vi "log analysis_gps.vi"() -> ()   [LabVIEW 2018] (continued)
02008000,d426,15824;INSUFFICIENT_OBS,NONE,0.000000000,0.000000000,0.000000000,0.0,0.000000000,0.000000000,\"\",0,0,0,0,00,00,00,00*bcb2c0dd\n\tsystem status\tnormal 2 28.100000 0 0\trobot status\t274.912306\t76.948987\t9.582700\t-0.292788\t1.088000\t-30.605308\t0.352000\t0.058000\n\t\n15:22:58.5\tlog_raw\tgps_raw\t#DUALANTENNAHEADINGA,USB3,0,49.0,FINESTEERING,2107,282196.500,02008000,d426,15824;SOL_COMPUTED,NARROW_FLOAT,-1.000000000,119.397575378,5.704736233,0.0,360.000000000,180.000000000,\"631T\",17,6,6,5,04,00,20,03*618b4b70\n\tsystem status\tnormal 2 28.000000 0 0\trobot status\t275.029815\t76.849491\t9.589700\t-0.210069\t0.973059\t-30.986366\t0.294000\t-0.025000\n\t\n15:22:59.0\tlog_raw\tgps_raw\t\tsystem status\tnormal 2 28.000000 0 0\trobot status\t275.145656\t76.747954\t9.596500\t-0.145332\t0.980754\t-31.500751\t0.356000\t0.072000\n\t\n15:22:59.5\tlog_raw\tgps_raw\t#DUALANTENNAHEADINGA,USB3,0,52.0,FINESTEERING,2107,282197.500,02008000,d426,15824;SOL_COMPUTED,NARROW_FLOAT,-1.000000000,59.046657562,-17.785888672,0.0,166.409759521,180.000000000,\"631T\",16,7,7,5,04,00,20,03*00118b7f\n\tsystem status\tnormal 2 28.000000 0 0\trobot status\t275.261842\t76.668742\t9.599000\t-0.003183\t0.966963\t-31.967987\t0.353000\t0.059000\n\t\n15:23:00.0\tlog_raw\tgps_raw\t#DUALANTENNAHEADINGA,USB3,0,52.0,FINESTEERING,2107,282198.000,02008000,d426,15824;SOL_COMPUTED,NARROW_FLOAT,-1.000000000,59.079334259,-18.122131348,0.0,167.196258545,180.000000000,\"631T\",16,7,7,5,04,00,20,03*485efbcb\n\tsystem status\tnormal 2 28.000000 0 0\trobot status\t275.377702\t76.588966\t9.600500\t-0.044192\t1.138417\t-32.357221\t0.252000\t-0.086000\n\t\n15:23:00.5\tlog_raw\tgps_raw\t#DUALANTENNAHEADINGA,USB3,0,50.0,FINESTEERING,2107,282198.500,02000000,d426,15824;SOL_COMPUTED,NARROW_FLOAT,-1.000000000,72.630279541,-6.125091553,0.0,217.219696045,180.000000000,\"631T\",16,8,8,5,04,00,20,03*03cea49d\n\tsystem status\tnormal 2 28.000000 0 0\trobot status\t275.489352\t76.505166\t9.604900\t-0.094622\t1.328061\t-32.726048\t0.293000\t-0.019000\n\t\n15:23:01.0\tlog_raw\tgps_raw\t#DUALANTENNAHEADINGA,USB3,0,50.0,FINESTEERING,2107,282199.000,02000000,d426,15824;SOL_COMPUTED,NARROW_FLOAT,-1.000000000,72.616973877,-5.097595215,0.0,218.517272949,180.000000000,\"631T\",18,8,8,5,04,00,20,03*278af582\n\tsystem status\tnormal 2 28.100000 0 0\trobot status\t275.601783\t76.419379\t9.608400\t-0.185416\t1.532796\t-32.964629\t0.298000\t-0.002000\n\t\n15:23:01.5\tlog_raw\tgps_raw\t#DUALANTENNAHEADINGA,USB3,0,51.0,FINESTEERING,2107,282199.500,02000000,d426,15824;INSUFFICIENT_OBS,NONE,0.000000000,0.000000000,0.000000000,0.0,0.000000000,0.000000000,\"\",0,0,0,0,00,00,00,00*6fb354b0\n\tsystem status\tnormal 2 28.000000 0 0\trobot status\t275.709417\t76.334818\t9.610400\t-0.145091\t1.698029\t-33.199566\t0.306000\t0.004000\n\t\n15:23:02.0\tlog_raw\tgps_raw\t\tsystem status\tnormal 2 28.100000 0 0\trobot status\t275.819505\t76.245723\t9.612400\t-0.060143\t1.689752\t-33.413572\t0.300000\t0.007000\n\t\n15:23:02.5\tlog_raw\tgps_raw\t#DUALANTENNAHEADINGA,USB3,0,51.5,FINESTEERING,2107,282200.500,02000000,d426,15824;INSUFFICIENT_OBS,NONE,0.000000000,0.000000000,0.000000000,0.0,0.000000000,0.000000000,\"\",0,0,0,0,00,00,00,00*ba5dc1a6\n\tsystem status\tnormal 2 28.100000 0 0\trobot status\t275.926001\t76.142312\t9.618400\t0.095795\t1.531020\t-33.633287\t0.295000\t0.013000\n\t\n15:23:03.0\tlog_raw\tgps_raw\t#DUALANTENNAHEADINGA,USB3,0,51.5,FINESTEERING,2107,282201.000,02000000,d426,15824;INSUFFICIENT_OBS,NONE,0.000000000,0.000000000,0.000000000,0.0,0.000000000,0.000000000,\"\",0,0,0,0,00,00,00,00*13cea2a1\n\tsystem status\tnormal 2 28.100000 0 0\trobot status\t276.031687\t76.036831\t9.624600\t0.090096\t1.284244\t-33.885924\t0.303000\t0.003000\n\t\n15:23:03.5\tlog_raw\tgps_raw\t#DUALANTENNAHEADINGA,USB3,0,53.0,FINESTEERING,2107,282201.500,02000000,d426,15824;INSUFFICIENT_OBS,NONE,0.000000000,0.000000000,0.000000000,0.0,0.000000000,0.000000000,\"\",0,0,0,0,00,00,00,00*311e64df\n\tsystem status\tnormal 2 28.100000 0 0\trobot status\t276.138696\t75.928855\t9.630700\t-0.035823\t1.113523\t-34.018971\t0.301000\t0.004000\n\t\n15:23:04.0\tlog_raw\tgps_raw\t#INSPVAXA,USB3,0,53.0,FINESTEERING,2107,282202.050,02000000,471d,15824;INS_ALIGNMENT_COMPLETE,INS_RTKFIXED,37.37081327952,126.72395394538,9.6368,22.3000,-0.2188,0.2169,0.0119,-0.186356861,0.873042918,124.050200417,0.5705,0.3686,0.6665,0.1331,0.1050,0.0820,0.1461,0.1508,4.9895,0f000001,0*b1c71fb3\n\tsystem status\tnormal 2 28.100000 0 0\trobot status\t276.261764\t75.807130\t9.636800\t-0.186357\t0.873043\t-34.050200\t0.298000\t0.025000\n\t\n15:23:04.5\tlog_raw\tgps_raw\t#DUALANTENNAHEADINGA,USB3,0,53.0,FINESTEERING,2107,282202.500,02000000,d426,15824;INSUFFICIENT_OBS,NONE,0.000000000,0.000000000,0.000000000,0.0,0.000000000,0.000000000,\"\",0,0,0,0,00,00,00,00*e4587ba4\n\tsystem status\tnormal 2 28.100000 0 0\trobot status\t276.364792\t75.742837\t9.636100\t-0.196635\t0.813843\t-34.065150\t0.302000\t0.016000\n\t\n15:23:05.0\tlog_raw\tgps_raw\t\tsystem status\tnormal 2 28.100000 0 0\trobot status\t276.481226\t75.668811\t9.635600\t-0.212412\t0.914728\t-33.926312\t0.295000\t0.037000\n\t\n15:23:05.5\tlog_raw\tgps_raw\t#DUALANTENNAHEADINGA,USB3,0,52.5,FINESTEERING,2107,282203.500,02000000,d426,15824;INSUFFICIENT_OBS,NONE,0.000000000,0.000000000,0.000000000,0.0,0.000000000,0.000000000,\"\",0,0,0,0,00,00,00,00*55500259\n\tsystem status\tnormal 2 28.000000 0 0\trobot status\t276.590081\t75.590259\t9.636200\t-0.255814\t1.160317\t-33.428711\t0.308000\t0.019000\n\t\n15:23:06.0\tlog_raw\tgps_raw\t#DUALANTENNAHEADINGA,USB3,0,52.5,FINESTEERING,2107,282204.000,02000000,d426,15824;INSUFFICIENT_OBS,NONE,0.000000000,0.000000000,0.000000000,0.0,0.000000000,0.000000000,\"\",0,0,0,0,00,00,00,00*8d3e59e9\n\tsystem status\tnormal 2 27.900000 0 0\trobot status\t276.699631\t75.510509\t9.636500\t-0.377307\t1.263158\t-32.842107\t0.247000\t0.122000\n\t\n15:23:06.5\tlog_raw\tgps_raw\t#DUALANTENNAHEADINGA,USB3,0,51.0,FINESTEERING,2107,282204.500,02000000,d426,15824;INSUFFICIENT_OBS,NONE,0.000000000,0.000000000,0.000000000,0.0,0.000000000,0.000000000,\"\",0,0,0,0,00,00,00,00*0f0729d4\n\tsystem status\tnormal 2 27.800000 0 0\trobot status\t276.809810\t75.428563\t9.637300\t-0.231259\t1.268189\t-32.036520\t0.321000\t-0.003000\n\t\n15:23:07.0\tlog_raw\tgps_raw\t#DUALANTENNAHEADINGA,USB3,0,51.0,FINESTEERING,2107,282205.000,02000000,d426,15824;INSUFFICIENT_OBS,NONE,0.000000000,0.000000000,0.000000000,0.0,0.000000000,0.000000000,\"\",0,0,0,0,00,00,00,00*a6944ad3\n\tsystem status\tnormal 2 27.800000 0 0\trobot status\t276.920112\t75.348048\t9.638800\t-0.239719\t1.316167\t-31.223244\t0.236000\t0.118000\n\t\n15:23:07.5\tlog_raw\tgps_raw\t#INSPVAXA,USB3,0,53.0,FINESTEERING,2107,282205.550,02000000,471d,15824;INS_ALIGNMENT_COMPLETE,INS_RTKFIXED,37.37080836161,126.72396276793,9.6416,22.3000,-0.1860,0.2071,0.0131,-0.386237620,1.395044510,120.415786575,0.4755,0.3044,0.5933,0.1227,0.0990,0.0774,0.1450,0.1497,4.9912,0f000001,0*671127a5\n\tsystem status\tnormal 2 27.800000 0 0\trobot status\t277.043251\t75.261292\t9.641600\t-0.386238\t1.395045\t-30.415787\t0.255000\t0.098000\n\t\n15:23:08.0\tlog_raw\tgps_raw\t#DUALANTENNAHEADINGA,USB3,0,53.0,FINESTEERING,2107,282206.000,02000000,d426,15824;INSUFFICIENT_OBS,NONE,0.000000000,0.000000000,0.000000000,0.0,0.000000000,0.000000000,\"\",0,0,0,0,00,00,00,00*e9703f6f\n\tsystem status\tnormal 2 27.900000 0 0\trobot status\t277.146093\t75.189189\t9.643900\t-0.464725\t1.386082\t-29.903743\t0.334000\t-0.013000\n\t\n15:23:08.5\tlog_raw\tgps_raw\t\tsystem status\tnormal 2 27.900000 0 0\trobot status\t277.259307\t75.112413\t9.646000\t-0.468117\t1.652568\t-29.339662\t0.270000\t0.070000\n\t\n15:23:09.0\tlog_raw\tgps_raw\t#INSPVAXA,USB3,0,52.0,FINESTEERING,2107,282207.050,02000000,471d,15824;INS_ALIGNMENT_COMPLETE,INS_RTKFIXED,37.37080624605,126.72396663060,9.6483,22.3000,-0.1799,0.2155,-0.0033,-0.382267918,1.666666307,118.913486054,0.4622,0.2990,0.5698,0.1222,0.0981,0.0770,0.1443,0.1494,4.9912,0f000001,0*412cbbed\n\tsystem status\tnormal 2 27.900000 0 0\trobot status\t277.385400\t75.026486\t9.648300\t-0.382268\t1.666666\t-28.913486\t0.315000\t-0.016000\n\t\n15:23:09.5\tlog_raw\tgps_raw\t#INSPVAXA,USB3,0,52.5,FINESTEERING,2107,282207.550,02000000,471d,15824;INS_ALIGNMENT_COMPLETE,INS_RTKFIXED,37.37080553452,126.72396795365,9.6521,22.3000,-0.1872,0.2206,-0.0051,-0.332963269,1.523153610,118.680008658,0.4622,0.2990,0.5698,0.1222,0.0981,0.0770,0.1443,0.1494,4.9912,0f000001,0*ceea6f3f\n\tsystem status\tnormal 2 28.000000 0 0\trobot status\t277.502593\t74.947513\t9.652100\t-0.332963\t1.523154\t-28.680009\t0.216000\t0.117000\n\t\n15:23:10.0\tlog_raw\tgps_raw\t#DUALANTENNAHEADINGA,USB3,0,52.5,FINESTEERING,2107,282208.000,02000000,d426,15824;INSUFFICIENT_OBS,NONE,0.000000000,0.000000000,0.000000000,0.0,0.000000000,0.000000000,\"\",0,0,0,0,00,00,00,00*6ec42887\n\tsystem status\tnormal 2 28.000000 0 0\trobot status\t277.607938\t74.876095\t9.655100\t-0.292418\t1.472958\t-28.591290\t0.334000\t-0.074000\n\t\n15:23:10.5\tlog_raw\tgps_raw\t\tsystem status\tnormal 2 28.000000 0 0\trobot status\t277.716428\t74.786283\t9.660500\t-0.341323\t1.522114\t-28.516894\t0.278000\t0.020000\n\t\n15:23:11.0\tlog_raw\tgps_raw\t\tsystem status\tnormal 2 28.100000 0 0\trobot status\t277.824920\t74.695483\t9.666100\t-0.489851\t1.492802\t-28.563133\t0.288000\t0.002000\n\t\n15:23:11.5\tlog_raw\tgps_raw\t#DUALANTENNAHEADINGA,USB3,0,53.0,FINESTEERING,2107,282209.500,02000000,d426,15824;SOL_COMPUTED,L1_FLOAT,-1.000000000,126.771110535,-42.657562256,0.0,360.000000000,180.000000000,\"631T\",15,6,6,5,04,00,20,03*5e6f8f1e\n\tsystem status\tnormal 2 28.100000 0 0\trobot status\t277.950579\t74.626425\t9.668500\t-0.427356\t1.503272\t-28.579089\t0.296000\t-0.011000\n\t\n15:23:12.0\tlog_raw\tgps_raw\t\tsystem status\tnormal 2 28.100000 0 0\trobot status\t278.077777\t74.556796\t9.671200\t-0.353609\t1.534540\t-28.611370\t0.297000\t-0.008000\n\t\n15:23:12.5\tlog_raw\tgps_raw\t#INSPVAXA,USB3,0,46.5,FINESTEERING,2107,282210.550,02000000,471d,15824;INS_ALIGNMENT_COMPLETE,INS_RTKFIXED,37.37080130132,126.72397594412,9.6761,22.3000,-0.1788,0.2268,0.0030,-0.286685420,1.503985922,118.659616564,0.4924,0.3183,0.5916,0.1238,0.0973,0.0785,0.1441,0.1495,4.9922,0f000001,0*a986a7a1\n\tsystem status\tnormal 2 28.100000 0 0\trobot status\t278.210376\t74.477669\t9.676100\t-0.286685\t1.503986\t-28.659617\t0.298000\t-0.010000\n\t\n15:23:13.0\tlog_raw\tgps_raw\t#INSPVAXA,USB3,0,46.5,FINESTEERING,2107,282211.050,02000000,471d,15824;INS_ALIGNMENT_COMPLETE,INS_RTKFIXED,37.37080065460,126.72397731700,9.6819,22.3000,-0.1828,0.2291,0.0069,-0.471563317,1.301185162,118.765096011,0.4785,0.3076,0.5799,0.1215,0.0954,0.0779,0.1439,0.1491,4.9928,0f000001,0*2dcee279\n\tsystem status\tnormal 2 28.000000 0 0\trobot status\t278.331984\t74.405889\t9.681900\t-0.471563\t1.301185\t-28.765096\t0.298000\t-0.016000\n\t\n15:23:13.5\tlog_raw\tgps_raw\t#INSPVAXA,USB3,0,49.5,FINESTEERING,2107,282211.550,02000000,471d,15824;INS_ALIGNMENT_COMPLETE,INS_RTKFIXED,37.37079998486,126.72397867623,9.6862,22.3000,-0.1762,0.2152,0.0021,-0.525326899,1.337901633,118.895801631,0.4785,0.3076,0.5799,0.1215,0.0954,0.0779,0.1439,0.1491,4.9928,0f000001,0*f623f6b1\n\tsystem status\tnormal 2 28.100000 0 0\trobot status\t278.452382\t74.331555\t9.686200\t-0.525327\t1.337902\t-28.895802\t0.297000\t-0.027000\n\t\n15:23:14.0\tlog_raw\tgps_raw\t\tsystem status\tnormal 2 28.100000 0 0\trobot status\t278.560279\t74.263479\t9.689600\t-0.578283\t1.310440\t-29.026777\t0.307000\t-0.012000\n\t\n15:23:14.5\tlog_raw\tgps_raw\t#INSPVAXA,USB3,0,48.0,FINESTEERING,2107,282212.550,02000000,471d,15824;INS_ALIGNMENT_COMPLETE,INS_RTKFIXED,37.37079858565,126.72398137805,9.6949,22.3000,-0.1865,0.2376,0.0037,-0.452411122,1.244077399,119.281089900,0.4696,0.3015,0.5709,0.1202,0.0946,0.0776,0.1439,0.1489,4.9934,0f000001,0*f2809ec3\n\tsystem status\tnormal 2 28.100000 0 0\trobot status\t278.691705\t74.176256\t9.694900\t-0.452411\t1.244077\t-29.281090\t0.298000\t-0.029000\n\t\n15:23:15.0\tlog_raw\tgps_raw\t#INSPVAXA,USB3,0,48.0,FINESTEERING,2107,282213.050,02000000,471d,15824;INS_ALIGNMENT_COMPLETE,INS_RTKFIXED,37.37079782312,126.72398277607,9.6996,22.3000,-0.1874,0.2360,0.0136,-0.341636601,1.253165011,119.484687507,0.4696,0.3015,0.5709,0.1202,0.0946,0.0776,0.1439,0.1489,4.9934,0f000001,0*32ae8dd5\n\tsystem status\tnormal 2 28.000000 0 0\trobot status\t278.815539\t74.091623\t9.699600\t-0.341637\t1.253165\t-29.484688\t0.300000\t-0.023000\n\t\n15:23:15.5\tlog_raw\tgps_raw\t#INSPVAXA,USB3,0,52.0,FINESTEERING,2107,282213.550,02000000,471d,15824;INS_ALIGNMENT_COMPLETE,INS_RTKFIXED,37.37079696943,126.72398406821,9.7061,22.3000,-0.1973,0.2288,0.0187,-0.230921805,1.180153263,119.768927864,0.4696,0.3015,0.5709,0.1202,0.0946,0.0776,0.1439,0.1489,4.9934,0f000001,0*21be5dd7\n\tsystem status\tnormal 2 28.000000 0 0\trobot status\t278.929995\t73.996872\t9.706100\t-0.230922\t1.180153\t-29.768928\t0.303000\t-0.009000\n\t\n15:23:16.0\tlog_raw\tgps_raw\t#INSPVAXA,USB3,0,52.0,FINESTEERING,2107,282214.050,02000000,471d,15824;INS_ALIGNMENT_COMPLETE,INS_RTKFIXED,37.37079609402,126.72398538509,9.7128,22.3000,-0.1984,0.2265,0.0093,-0.318894921,1.159811562,120.132243890,0.4696,0.3015,0.5709,0.1202,0.0946,0.0776,0.1439,0.1489,4.9934,0f000001,0*fc389eb4\n\tsystem status\tnormal 2 28.100000 0 0\trobot status\t279.046642\t73.899711\t9.712800\t-0.318895\t1.159812\t-30.132244\t0.277000\t-0.051000\n\t\n15:23:16.5\tlog_raw\tgps_raw\t\tsystem status\tnormal 2 28.000000 0 0\trobot status\t279.147927\t73.812646\t9.718900\t-0.463860\t1.163408\t-30.444630\t0.301000\t-0.026000\n\t\n15:23:17.0\tlog_raw\tgps_raw\t#INSPVAXA,USB3,0,52.0,FINESTEERING,2107,282215.050,02000000,471d,15824;INS_ALIGNMENT_COMPLETE,INS_RTKFIXED,37.37079433087,126.72398790668,9.7264,22.3000,-0.2059,0.2196,0.0017,-0.257763882,1.185688863,120.911498528,0.5642,0.3665,0.6560,0.1320,0.1043,0.0817,0.1458,0.1507,4.9969,0f000001,0*cb6b0c5a\n\tsystem status\tnormal 2 28.000000 0 0\trobot status\t279.270000\t73.704021\t9.726400\t-0.257764\t1.185689\t-30.911499\t0.331000\t0.039000\n\t\n15:23:17.5\tlog_raw\tgps_raw\t#INSPVAXA,USB3,0,51.0,FINESTEERING,2107,282215.550,02000000,471d,15824;INS_ALIGNMENT_COMPLETE,INS_RTKFIXED,37.37079367366,126.72398934399,9.7308,22.3000,-0.1996,0.2242,0.0120,-0.145309566,1.145371194,121.351414848,0.5642,0.3665,0.6560,0.1320,0.1043,0.0817,0.1458,0.1507,4.9969,0f000001,0*eab453aa\n\tsystem status\tnormal 2 28.000000 0 0\trobot status\t279.397315\t73.631077\t9.730800\t-0.145310\t1.145371\t-31.351415\t0.343000\t0.047000\n\t\n15:23:18.0\tlog_raw\tgps_raw\t#INSPVAXA,USB3,0,50.0,FINESTEERING,2107,282216.050,02008000,471d,15824;INS_ALIGNMENT_COMPLETE,INS_RTKFIXED,37.37079301498,126.72399074721,9.7351,22.3000,-0.2016,0.2239,0.0141,-0.200785279,1.162503620,121.722794866,0.5181,0.3306,0.6284,0.1253,0.0993,0.0793,0.1452,0.1498,4.9985,0f000001,0*bb6b6e1a\n\tsystem status\tnormal 2 28.100000 0 0\trobot status\t279.521610\t73.557970\t9.735100\t-0.200785\t1.162504\t-31.722795\t0.350000\t0.062000\n\t\n15:23:18.5\tlog_raw\tgps_raw\t#INSPVAXA,USB3,0,50.0,FINESTEERING,2107,282216.550,02008000,471d,15824;INS_ALIGNMENT_COMPLETE,INS_RTKFIXED,37.37079227472,126.72399206413,9.7382,22.3000,-0.1946,0.2230,0.0198,-0.317684959,1.282586608,122.063744608,0.5181,0.3306,0.6284,0.1253,0.0993,0.0793,0.1452,0.1498,4.9985,0f000001,0*e6f737e3\n\tsystem status\tnormal 2 28.100000 0 0\trobot status\t279.638260\t73.475808\t9.738200\t-0.317685\t1.282587\t-32.063745\t0.299000\t-0.007000\n\t\n15:23:19.0\tlog_raw\tgps_raw\t#INSPVAXA,USB3,0,50.0,FINESTEERING,2107,282217.050,02008000,471d,15824;INS_ALIGNMENT_COMPLETE,INS_RTKFIXED,37.37079150006,126.72399338506,9.7418,22.3000,-0.1973,0.2143,0.0166,-0.258493900,1.347892765,122.299122592,0.4919,0.3126,0.6073,0.1228,0.0982,0.0779,0.1450,0.1495,4.9999,0f000001,0*de2ea87f\n\tsystem status\tnormal 2 28.100000 0 0\trobot status\t279.755266\t73.389829\t9.741800\t-0.258494\t1.347893\t-32.299123\t0.297000\t-0.005000\n\t\n15:23:19.5\tlog_raw\tgps_raw\t\tsystem status\tnormal 2 28.100000 0 0\trobot status\t279.855684\t73.313958\t9.747600\t-0.193916\t1.492610\t-32.596087\t0.298000\t-0.002000\n\t\n15:23:20.0\tlog_raw\tgps_raw\t\tsystem status\tnormal 2 28.000000 0 0\trobot status\t279.966679\t73.228541\t9.754600\t-0.196447\t1.616666\t-32.901459\t0.292000\t-0.010000\n\t\n15:23:20.5\tlog_raw\tgps_raw\t#INSPVAXA,USB3,0,51.5,FINESTEERING,2107,282218.550,02008000,471d,15824;INS_ALIGNMENT_COMPLETE,INS_RTKFIXED,37.37078915904,126.72399716309,9.7610,22.3000,-0.2130,0.2098,0.0170,-0.292581924,1.665037995,123.167578818,0.4769,0.3037,0.5912,0.1221,0.0981,0.0771,0.1448,0.1493,5.0010,0f000001,0*5a89842f\n\tsystem status\tnormal 2 28.100000 0 0\trobot status\t280.089918\t73.130001\t9.761000\t-0.292582\t1.665038\t-33.167579\t0.297000\t-0.001000\n\t\n15:23:21.0\tlog_raw\tgps_raw\t#INSPVAXA,USB3,0,51.5,FINESTEERING,2107,282219.050,02008000,471d,15824;INS_ALIGNMENT_COMPLETE,INS_RTKFIXED,37.37078832063,126.72399842807,9.7659,22.3000,-0.2077,0.2129,0.0166,-0.240249053,1.576876220,123.403306266,0.4687,0.2996,0.5787,0.1217,0.0981,0.0767,0.1445,0.1492,5.0017,0f000001,0*d445f717\n\tsystem status\tnormal 2 28.100000 0 0\trobot status\t280.201968\t73.036946\t9.765900\t-0.240249\t1.576876\t-33.403306\t0.300000\t0.000000\n\t\n15:23:21.5\tlog_raw\tgps_raw\t#INSPVAXA,USB3,0,52.5,FINESTEERING,2107,282219.550,02008000,471d,15824;INS_ALIGNMENT_COMPLETE,INS_RTKFIXED,37.37078751914,126.72399965144,9.7712,22.3000,-0.2065,0.2085,0.0140,-0.281116396,1.447393421,123.657865027,0.4687,0.2996,0.5787,0.1217,0.0981,0.0767,0.1445,0.1492,5.0017,0f000001,0*13bb7dd6\n\tsystem status\tnormal 2 28.000000 0 0\trobot status\t280.310332\t72.947989\t9.771200\t-0.281116\t1.447393\t-33.657865\t0.300000\t0.003000\n\t\n15:23:22.0\tlog_raw\tgps_raw\t#INSPVAXA,USB3,0,52.5,FINESTEERING,2107,282220.050,02008000,471d,15824;INS_ALIGNMENT_COMPLETE,INS_RTKFIXED,37.37078669426,126.72400086844,9.7773,22.3000,-0.1998,0.2016,0.0200,-0.389870934,1.544632790,123.892841428,0.4687,0.2996,0.5787,0.1217,0.0981,0.0767,0.1445,0.1492,5.0017,0f000001,0*0724934d\n\tsystem status\tnormal 2 28.100000 0 0\trobot status\t280.418132\t72.856437\t9.777300\t-0.389871\t1.544633\t-33.892841\t0.298000\t0.008000\n\t\n15:23:22.5\tlog_raw\tgps_raw\t#INSPVAXA,USB3,0,45.0,FINESTEERING,2107,282220.550,02000000,471d,15824;INS_ALIGNMENT_COMPLETE,INS_RTKFIXED,37.37078572061,126.72400205426,9.7874,22.3000,-0.2160,0.2146,0.0148,-0.304638903,1.496803288,124.054451305,0.4687,0.2996,0.5787,0.1217,0.0981,0.0767,0.1445,0.1492,5.0017,0f000001,0*4ea05ecc\n\tsystem status\tnormal 2 28.100000 0 0\trobot status\t280.523169\t72.748373\t9.787400\t-0.304639\t1.496803\t-34.054451\t0.302000\t0.004000\n\t\n15:23:23.0\tlog_raw\tgps_raw\t#INSPVAXA,USB3,0,45.0,FINESTEERING,2107,282221.050,02000000,471d,15824;INS_ALIGNMENT_COMPLETE,INS_RTKFIXED,37.37078472745,126.72400323556,9.7963,22.3000,-0.2252,0.2194,0.0154,-0.213568919,1.398343739,124.133980325,0.4687,0.2996,0.5787,0.1217,0.0981,0.0767,0.1445,0.1492,5.0017,0f000001,0*532042ec\n\tsystem status\tnormal 2 28.100000 0 0\trobot status\t280.627807\t72.638144\t9.796300\t-0.213569\t1.398344\t-34.133980\t0.299000\t0.014000\n\t\n15:23:23.5\tlog_raw\tgps_raw\t#INSPVAXA,USB3,0,51.5,FINESTEERING,2107,282221.550,02000000,471d,15824;INS_ALIGNMENT_COMPLETE,INS_RTKFIXED,37.37078368778,126.72400445240,9.8057,22.3000,-0.2341,0.2209,0.0324,-0.018062526,1.300633595,124.151210863,0.4687,0.2996,0.5787,0.1217,0.0981,0.0767,0.1445,0.1492,5.0017,0f000001,0*d5cded7b\n\tsystem status\tnormal 2 28.000000 0 0\trobot status\t280.735593\t72.522753\t9.805700\t-0.018063\t1.300634\t-34.151211\t0.299000\t0.020000\n\t\n15:23:24.0\tlog_raw\tgps_raw\t#INSPVAXA,USB3,0,51.5,FINESTEERING,2107,282222.050,02000000,471d,15824;INS_ALIGNMENT_COMPLETE,INS_RTKFIXED,37.37078266162,126.72400570863,9.8159,22.3000,-0.2293,0.2203,0.0286,-0.177364447,1.182183127,124.095380159,0.5655,0.3677,0.6592,0.1343,0.1069,0.0811,0.1457,0.1508,5.0028,0f000001,0*1d515c3b\n\tsystem status\tnormal 2 28.000000 0 0\trobot status\t280.846868\t72.408862\t9.815900\t-0.177364\t1.182183\t-34.095380\t0.310000\t0.021000\n\t\n15:23:24.5\tlog_raw\tgps_raw\t#INSPVAXA,USB3,0,52.0,FINESTEERING,2107,282222.550,02000000,471d,15824;INS_ALIGNMENT_COMPLETE,INS_RTKFIXED,37.37078201526,126.72400713650,9.8181,22.3000,-0.2189,0.2044,0.0167,-0.239686925,1.045245044,123.863741135,0.5655,0.3677,0.6592,0.1343,0.1069,0.0811,0.1457,0.1508,5.0028,0f000001,0*9d8dd707\n\tsystem status\tnormal 2 28.000000 0 0\trobot status\t280.973346\t72.337121\t9.818100\t-0.239687\t1.045245\t-33.863741\t0.216000\t0.162000\n\t\n15:23:25.0\tlog_raw\tgps_raw\t#INSPVAXA,USB3,0,52.0,FINESTEERING,2107,282223.050,02000000,471d,15824;INS_ALIGNMENT_COMPLETE,INS_RTKFIXED,37.37078138218,126.72400846731,9.8199,22.3000,-0.2177,0.1996,0.0188,-0.144202843,1.121525384,123.301599310,0.5655,0.3677,0.6592,0.1343,0.1069,0.0811,0.1457,0.1508,5.0028,0f000001,0*4658464e\n\tsystem status\tnormal 2 27.900000 0 0\trobot status\t281.091227\t72.266855\t9.819900\t-0.144203\t1.121525\t-33.301599\t0.293000\t0.053000\n\t\n15:23:25.5\tlog_raw\tgps_raw\t#INSPVAXA,USB3,0,52.0,FINESTEERING,2107,282223.550,02000000,471d,15824;INS_ALIGNMENT_COMPLETE,INS_RTKFIXED,37.37078042542,126.72400959885,9.8298,22.3000,-0.1980,0.1883,0.0199,0.083241737,1.323181933,122.442356839,0.5655,0.3677,0.6592,0.1343,0.1069,0.0811,0.1457,0.1508,5.0028,0f000001,0*8c550850\n\tsystem status\tnormal 2 27.800000 0 0\trobot status\t281.191457\t72.160666\t9.829800\t0.083242\t1.323182\t-32.442357\t0.225000\t0.116000\n\t\n15:23:26.0\tlog_raw\tgps_raw\t#INSPVAXA,USB3,0,52.0,FINESTEERING,2107,282224.050,02000000,471d,15824;INS_ALIGNMENT_COMPLETE,INS_RTKFIXED,37.37077948836,126.72401076262,9.8410,22.3000,-0.2038,0.2000,0.0255,0.037457122,1.616174410,121.334966329,0.5655,0.3677,0.6592,0.1343,0.1069,0.0811,0.1457,0.1508,5.0028,0f000001,0*1dc4c535\n\tsystem status\tnormal 2 27.800000 0 0\trobot status\t281.294542\t72.056663\t9.841000\t0.037457\t1.616174\t-31.334966\t0.235000\t0.135000\n\t\n15:23:26.5\tlog_raw\tgps_raw\t#INSPVAXA,USB3,0,53.0,FINESTEERING,2107,282224.550,02000000,471d,15824;INS_ALIGNMENT_COMPLETE,INS_RTKFIXED,37.37077854921,126.72401195388,9.8525,22.3000,-0.2034,0.2018,0.0231,0.005685639,1.610626959,120.264541243,0.5655,0.3677,0.6592,0.1343,0.1069,0.0811,0.1457,0.1508,5.0028,0f000001,0*90090751\n\tsystem status\tnormal 2 27.800000 0 0\trobot status\t281.400062\t71.952429\t9.852500\t0.005686\t1.610627\t-30.264541\t0.243000\t0.132000\n\t\n15:23:27.0\tlog_raw\tgps_raw\t#INSPVAXA,USB3,0,53.0,FINESTEERING,2107,282225.050,02000000,471d,15824;INS_ALIGNMENT_COMPLETE,INS_RTKFIXED,37.37077766145,126.72401317567,9.8633,22.3000,-0.2009,0.2209,0.0247,-0.192396038,1.572189477,119.250218807,0.6084,0.3900,0.7185,0.1389,0.1090,0.0824,0.1462,0.1512,5.0046,0f000001,0*0ea2a365\n\tsystem status\tnormal 2 27.700000 0 0\trobot status\t281.508286\t71.853897\t9.863300\t-0.192396\t1.572189\t-29.250219\t0.373000\t-0.059000\n\t\n15:23:27.5\tlog_raw\tgps_raw\t#INSPVAXA,USB3,0,52.5,FINESTEERING,2107,282225.550,02000000,471d,15824;INS_ALIGNMENT_COMPLETE,INS_RTKFIXED,37.37077734941,126.72401466448,9.8621,22.3000,-0.1997,0.2260,0.0207,-0.108448502,1.711031011,118.230862766,0.6084,0.3900,0.7185,0.1389,0.1090,0.0824,0.1462,0.1512,5.0046,0f000001,0*0e52b076\n\tsystem status\tnormal 2 27.700000 0 0\trobot status\t281.640162\t71.819261\t9.862100\t-0.108449\t1.711031\t-28.230863\t0.328000\t0.006000\n\t\n15:23:28.0\tlog_raw\tgps_raw\t#INSPVAXA,USB3,0,48.5,FINESTEERING,2107,282226.050,02000000,471d,15824;INS_ALIGNMENT_COMPLETE,INS_RTKFIXED,37.37077704777,126.72401614595,9.8618,22.3000,-0.1720,0.2084,0.0247,-0.161231391,1.488834735,117.043709795,0.5373,0.3399,0.6690,0.1307,0.1036,0.0789,0.1454,0.1502,5.0054,0f000001,0*01dce4f3\n\tsystem status\tnormal 2 27.700000 0 0\trobot status\t281.771388\t71.785780\t9.861800\t-0.161231\t1.488835\t-27.043710\t0.291000\t0.030000\n\t\n15:23:28.5\tlog_raw\tgps_raw\t\tsystem status\tnormal 2 27.900000 0 0\trobot status\t281.893755\t71.724784\t9.862200\t-0.244817\t1.370879\t-26.237375\t0.290000\t0.014000\n\t\n15:23:29.0\tlog_raw\tgps_raw\t#INSPVAXA,USB3,0,48.5,FINESTEERING,2107,282227.050,02000000,471d,15824;INS_ALIGNMENT_COMPLETE,INS_RTKFIXED,37.37077593278,126.72401891596,9.8631,22.3000,-0.1697,0.2262,0.0181,-0.178975170,1.493639019,115.812677176,0.5005,0.3171,0.6343,0.1279,0.1027,0.0771,0.1451,0.1499,5.0056,0f000001,0*b5f48b56\n\tsystem status\tnormal 2 27.900000 0 0\trobot status\t282.016751\t71.662025\t9.863100\t-0.178975\t1.493639\t-25.812677\t0.230000\t0.093000\n\t\n15:23:29.5\tlog_raw\tgps_raw\t#INSPVAXA,USB3,0,51.0,FINESTEERING,2107,282227.550,02000000,471d,15824;INS_ALIGNMENT_COMPLETE,INS_RTKFIXED,37.37077534199,126.72402027291,9.8655,22.3000,-0.1792,0.2154,0.0259,-0.205196219,1.587681370,115.700553222,0.5005,0.3171,0.6343,0.1279,0.1027,0.0771,0.1451,0.1499,5.0056,0f000001,0*9a4eb5a2\n\tsystem status\tnormal 2 28.000000 0 0\trobot status\t282.136948\t71.596452\t9.865500\t-0.205196\t1.587681\t-25.700553\t0.237000\t0.088000\n\t\n15:23:30.0\tlog_raw\tgps_raw\t#INSPVAXA,USB3,0,51.0,FINESTEERING,2107,282228.050,02000000,471d,15824;INS_ALIGNMENT_COMPLETE,INS_RTKFIXED,37.37077473925,126.72402159293,9.8669,22.3000,-0.1676,0.2065,0.0190,-0.168899804,1.509556154,115.821588566,0.4803,0.3065,0.6087,0.1271,0.1026,0.0763,0.1447,0.1496,5.0053,0f000001,0*25784804\n\tsystem status\tnormal 2 28.100000 0 0\trobot status\t282.253873\t71.529553\t9.866900\t-0.168900\t1.509556\t-25.821589\t0.293000\t-0.031000\n\t\n15:23:30.5\tlog_raw\tgps_raw\t#INSPVAXA,USB3,0,52.5,FINESTEERING,2107,282228.550,02000000,471d,15824;INS_ALIGNMENT_COMPLETE,INS_RTKFIXED,37.37077412906,126.72402288572,9.8668,22.3000,-0.1602,0.2130,0.0258,-0.196596636,1.388177172,115.979386072,0.4803,0.3065,0.6087,0.1271,0.1026,0.0763,0.1447,0.1496,5.0053,0f000001,0*cbeb8b2e\n\tsystem status\tnormal 2 28.100000 0 0\trobot status\t282.368386\t71.461828\t9.866800\t-0.196597\t1.388177\t-25.979386\t0.298000\t-0.042000\n\t\n15:23:31.0\tlog_raw\tgps_raw\t#INSPVAXA,USB3,0,50.5,FINESTEERING,2107,282229.050,02000000,471d,15824;INS_ALIGNMENT_COMPLETE,INS_RTKFIXED,37.37077350628,126.72402417744,9.8684,22.3000,-0.1816,0.2229,0.0203,-0.296207057,1.402486363,116.142608902,0.4697,0.3022,0.5898,0.1268,0.1020,0.0761,0.1442,0.1494,5.0046,0f000001,0*7993bda1\n\tsystem status\tnormal 2 28.000000 0 0\trobot status\t282.482805\t71.392705\t9.868400\t-0.296207\t1.402486\t-26.142609\t0.298000\t-0.037000\n\t\n15:23:31.5\tlog_raw\tgps_raw\t#INSPVAXA,USB3,0,50.5,FINESTEERING,2107,282229.550,02000000,471d,15824;INS_ALIGNMENT_COMPLETE,INS_RTKFIXED,37.37077278657,126.72402567791,9.8734,22.3000,-0.1941,0.2532,0.0237,-0.163503095,1.302197748,116.467398077,0.4697,0.3022,0.5898,0.1268,0.1020,0.0761,0.1442,0.1494,5.0046,0f000001,0*18de387b\n\tsystem status\tnormal 2 28.000000 0 0\trobot status\t282.615714\t71.312823\t9.873400\t-0.163503\t1.302198\t-26.467398\t0.308000\t-0.034000\n\t\n15:23:32.0\tlog_raw\tgps_raw\t#INSPVAXA,USB3,0,50.5,FINESTEERING,2107,282230.050,02000000,471d,15824;INS_ALIGNMENT_COMPLETE,INS_RTKFIXED,37.37077205146,126.72402713587,9.8769,22.3000,-0.1969,0.2300,0.0189,-0.143209861,1.267665510,116.875874478,0.4697,0.3022,0.5898,0.1268,0.1020,0.0761,0.1442,0.1494,5.0046,0f000001,0*6a8b4120\n\tsystem status\tnormal 2 28.000000 0 0\trobot status\t282.744857\t71.231233\t9.876900\t-0.143210\t1.267666\t-26.875874\t0.289000\t-0.056000\n\t\n15:23:32.5\tlog_raw\tgps_raw\t\tsystem status\tnormal 2 28.000000 0 0\trobot status\t282.858868\t71.138125\t9.883400\t-0.290779\t1.215600\t-27.642296\t0.368000\t0.050000\n\t\n15:23:33.0\tlog_raw\tgps_raw\t#INSPVAXA,USB3,0,50.5,FINESTEERING,2107,282231.050,02000000,471d,15824;INS_ALIGNMENT_COMPLETE,INS_RTKFIXED,37.37077037953,126.72402966350,9.8905,22.3000,-0.1831,0.2077,0.0203,-0.481877841,1.390379497,118.801399041,0.5188,0.3394,0.6182,0.1322,0.1054,0.0787,0.1443,0.1499,5.0038,0f000001,0*a6adcd9b\n\tsystem status\tnormal 2 27.900000 0 0\trobot status\t282.968751\t71.045667\t9.890500\t-0.481878\t1.390379\t-28.801399\t0.310000\t-0.010000\n\t\n15:23:33.5\tlog_raw\tgps_raw\t#INSPVAXA,USB3,0,51.0,FINESTEERING,2107,282231.550,02000000,471d,15824;INS_ALIGNMENT_COMPLETE,INS_RTKFIXED,37.37076971531,126.72403108088,9.8920,22.3000,-0.2013,0.2070,0.0109,-0.551553251,1.424964992,120.007848450,0.5188,0.3394,0.6182,0.1322,0.1054,0.0787,0.1443,0.1499,5.0038,0f000001,0*6cb6a544\n\tsystem status\tnormal 2 27.800000 0 0\trobot status\t283.094300\t70.971945\t9.892000\t-0.551553\t1.424965\t-30.007848\t0.282000\t-0.066000\n\t\n15:23:34.0\tlog_raw\tgps_raw\t\tsystem status\tnormal 2 27.800000 0 0\trobot status\t283.219222\t70.892043\t9.893500\t-0.314120\t1.375638\t-31.158834\t0.298000\t-0.058000\n\t\n15:23:34.5\tlog_raw\tgps_raw\t#INSPVAXA,USB3,0,48.0,FINESTEERING,2107,282232.550,02000000,471d,15824;INS_ALIGNMENT_COMPLETE,INS_RTKFIXED,37.37076823474,126.72403383781,9.8941,22.3000,-0.2085,0.2221,0.0077,-0.388348000,1.567603173,122.220869009,0.4952,0.3205,0.5986,0.1271,0.0996,0.0779,0.1435,0.1490,5.0025,0f000001,0*80bf9f92\n\tsystem status\tnormal 2 27.800000 0 0\trobot status\t283.338504\t70.807616\t9.894100\t-0.388348\t1.567603\t-32.220869\t0.351000\t0.038000\n\t\n15:23:35.0\tlog_raw\tgps_raw\t\tsystem status\tnormal 2 27.900000 0 0\trobot status\t283.458018\t70.716066\t9.894700\t-0.430593\t1.507673\t-33.146844\t0.247000\t-0.105000\n\t\n15:23:35.5\tlog_raw\tgps_raw\t#INSPVAXA,USB3,0,50.0,FINESTEERING,2107,282233.550,02000000,471d,15824;INS_ALIGNMENT_COMPLETE,INS_RTKFIXED,37.37076641843,126.72403639264,9.9004,22.3000,-0.2178,0.2114,0.0096,-0.342808402,1.379099654,123.844356856,0.4952,0.3205,0.5986,0.1271,0.0996,0.0779,0.1435,0.1490,5.0025,0f000001,0*b00cd8f2\n\tsystem status\tnormal 2 27.900000 0 0\trobot status\t283.564807\t70.606026\t9.900400\t-0.342808\t1.379100\t-33.844357\t0.349000\t0.040000\n\t\n15:23:36.0\tlog_raw\tgps_raw\t#INSPVAXA,USB3,0,50.0,FINESTEERING,2107,282234.050,02000000,471d,15824;INS_ALIGNMENT_COMPLETE,INS_RTKFIXED,37.37076539646,126.72403759594,9.9065,22.3000,-0.2225,0.2060,0.0095,-0.323054638,1.365837565,124.363784031,0.4952,0.3205,0.5986,0.1271,0.0996,0.0779,0.1435,0.1490,5.0025,0f000001,0*63b70899\n\tsystem status\tnormal 2 28.000000 0 0\trobot status\t283.671393\t70.492599\t9.906500\t-0.323055\t1.365838\t-34.363784\t0.357000\t0.078000\n\t\n15:23:36.5\tlog_raw\tgps_raw\t\tsystem status\tnormal 2 28.000000 0 0\trobot status\t283.776449\t70.376829\t9.912800\t-0.212693\t1.379976\t-34.712636\t0.281000\t-0.020000\n\t\n15:23:37.0\tlog_raw\tgps_raw\t#INSPVAXA,USB3,0,52.5,FINESTEERING,2107,282235.050,02000000,471d,15824;INS_ALIGNMENT_COMPLETE,INS_RTKFIXED,37.37076332295,126.72403997269,9.9185,22.3000,-0.2405,0.1895,0.0090,-0.183163482,1.364210608,124.971240350,0.5787,0.3754,0.6724,0.1350,0.1055,0.0817,0.1450,0.1501,5.0042,0f000001,0*0695c6fe\n\tsystem status\tnormal 2 28.100000 0 0\trobot status\t283.881922\t70.262464\t9.918500\t-0.183163\t1.364211\t-34.971240\t0.287000\t-0.008000\n\t\n15:23:37.5\tlog_raw\tgps_raw\t#INSPVAXA,USB3,0,52.5,FINESTEERING,2107,282235.550,02000000,471d,15824;INS_ALIGNMENT_COMPLETE,INS_RTKFIXED,37.37076275238,126.72404129303,9.9173,22.3000,-0.2324,0.1950,0.0071,-0.186698701,1.433095959,125.178228053,0.5787,0.3754,0.6724,0.1350,0.1055,0.0817,0.1450,0.1501,5.0042,0f000001,0*22a772a5\n\tsystem status\tnormal 2 28.000000 0 0\trobot status\t283.998875\t70.199136\t9.917300\t-0.186699\t1.433096\t-35.178228\t0.300000\t0.030000\n\t\n15:23:38.0\tlog_raw\tgps_raw\t#INSPVAXA,USB3,0,51.0,FINESTEERING,2107,282236.050,02000000,471d,15824;INS_ALIGNMENT_COMPLETE,INS_RTKFIXED,37.37076213061,126.72404264687,9.9162,22.3000,-0.2356,0.2149,0.0160,-0.109376323,1.538913747,125.183228459,0.5240,0.3345,0.6382,0.1270,0.0999,0.0792,0.1443,0.1492,5.0048,0f000001,0*e39a076f\n\tsystem status\tnormal 2 28.100000 0 0\trobot status\t284.118796\t70.130125\t9.916200\t-0.109376\t1.538914\t-35.183228\t0.298000\t0.031000\n\t\n15:23:38.5\tlog_raw\tgps_raw\t\tsystem status\tnormal 2 28.000000 0 0\trobot status\t284.240865\t70.041543\t9.917400\t-0.163307\t1.553018\t-35.162946\t0.308000\t0.016000\n\t\n15:23:39.0\tlog_raw\tgps_raw\t#INSPVAXA,USB3,0,51.0,FINESTEERING,2107,282237.050,02000000,471d,15824;INS_ALIGNMENT_COMPLETE,INS_RTKFIXED,37.37076053615,126.72404538521,9.9185,22.3000,-0.2398,0.2523,0.0058,-0.149955432,1.536125900,125.085519397,0.4941,0.3144,0.6129,0.1240,0.0987,0.0779,0.1441,0.1488,5.0061,0f000001,0*b0cbabaf\n\tsystem status\tnormal 2 28.000000 0 0\trobot status\t284.361354\t69.953156\t9.918500\t-0.149955\t1.536126\t-35.085519\t0.336000\t-0.012000\n\t\n15:23:39.5\tlog_raw\tgps_raw\t\tsystem status\tnormal 2 28.000000 0 0\trobot status\t284.476369\t69.863512\t9.923100\t-0.094683\t1.411903\t-34.808962\t0.374000\t-0.100000\n\t\n15:23:40.0\tlog_raw\tgps_raw\t#INSPVAXA,USB3,0,49.0,FINESTEERING,2107,282238.050,02000000,471d,15824;INS_ALIGNMENT_COMPLETE,INS_RTKFIXED,37.37075892495,126.72404799622,9.9275,22.3000,-0.2194,0.2349,0.0204,-0.036624693,1.339643543,124.302497248,0.4765,0.3044,0.5938,0.1228,0.0987,0.0772,0.1439,0.1487,5.0076,0f000001,0*d84ea5b6\n\tsystem status\tnormal 2 27.900000 0 0\trobot status\t284.592633\t69.774330\t9.927500\t-0.036625\t1.339644\t-34.302497\t0.273000\t0.059000\n\t\n15:23:40.5\tlog_raw\tgps_raw\t\tsystem status\tnormal 2 27.900000 0 0\trobot status\t284.707702\t69.684435\t9.930500\t-0.050498\t1.305539\t-33.760020\t0.291000\t0.040000\n\t\n15:23:41.0\tlog_raw\tgps_raw\t#INSPVAXA,USB3,0,49.0,FINESTEERING,2107,282239.050,02000000,471d,15824;INS_ALIGNMENT_COMPLETE,INS_RTKFIXED,37.37075731633,126.72405060135,9.9337,22.3000,-0.2234,0.2366,0.0085,-0.038602813,1.211050362,123.083406673,0.4672,0.3000,0.5797,0.1224,0.0986,0.0769,0.1436,0.1486,5.0092,0f000001,0*2a044e17\n\tsystem status\tnormal 2 27.900000 0 0\trobot status\t284.823391\t69.595790\t9.933700\t-0.038603\t1.211050\t-33.083407\t0.284000\t0.037000\n\t\n15:23:41.5\tlog_raw\tgps_raw\t\tsystem status\tnormal 2 27.800000 0 0\trobot status\t284.938172\t69.511116\t9.935100\t-0.087979\t1.240671\t-32.330627\t0.240000\t0.104000\n\t\n15:23:42.0\tlog_raw\tgps_raw\t#INSPVAXA,USB3,0,52.5,FINESTEERING,2107,282240.050,02000000,471d,15824;INS_ALIGNMENT_COMPLETE,INS_RTKFIXED,37.37075580155,126.72405321567,9.9361,22.3000,-0.2036,0.2395,0.0145,-0.175150317,1.281192873,121.711657184,0.4620,0.2982,0.5691,0.1221,0.0979,0.0769,0.1433,0.1484,5.0109,0f000001,0*31735912\n\tsystem status\tnormal 2 27.900000 0 0\trobot status\t285.054963\t69.427665\t9.936100\t-0.175150\t1.281193\t-31.711657\t0.227000\t0.112000\n\t\n15:23:42.5\tlog_raw\tgps_raw\t#INSPVAXA,USB3,0,52.0,FINESTEERING,2107,282240.550,02000000,471d,15824;INS_ALIGNMENT_COMPLETE,INS_RTKFIXED,37.37075505273,126.72405453213,9.9380,22.3000,-0.2095,0.2475,0.0059,-0.133753229,1.305172300,121.169613627,0.4620,0.2982,0.5691,0.1221,0.0979,0.0769,0.1433,0.1484,5.0109,0f000001,0*e864ebce\n\tsystem status\tnormal 2 27.900000 0 0\trobot status\t285.171573\t69.344553\t9.938000\t-0.133753\t1.305172\t-31.169614\t0.365000\t-0.090000\n\t\n15:23:43.0\tlog_raw\tgps_raw\t\tsystem status\tnormal 2 27.900000 0 0\trobot status\t285.288500\t69.261504\t9.940300\t-0.030325\t1.290477\t-30.615735\t0.394000\t-0.140000\n\t\n15:23:43.5\tlog_raw\tgps_raw\t\tsystem status\tnormal 2 27.900000 0 0\trobot status\t285.405117\t69.178632\t9.944700\t-0.092254\t1.253355\t-30.224738\t0.257000\t0.056000\n\t\n15:23:44.0\tlog_raw\tgps_raw\t\tsystem status\tnormal 2 28.000000 0 0\trobot status\t285.524434\t69.093762\t9.949700\t-0.145884\t1.178082\t-29.952582\t0.249000\t0.087000\n\t\n15:23:44.5\tlog_raw\tgps_raw\t\tsystem status\tnormal 2 28.000000 0 0\trobot status\t285.650277\t68.993089\t9.956200\t-0.075406\t1.044485\t-29.759550\t0.340000\t-0.073000\n\t\n15:23:45.0\tlog_raw\tgps_raw\t#INSPVAXA,USB3,0,48.5,FINESTEERING,2107,282243.050,02000000,471d,15824;INS_ALIGNMENT_COMPLETE,INS_RTKFIXED,37.37075099194,126.72406136178,9.9623,22.3000,-0.1962,0.2522,0.0127,-0.046095058,0.957232384,119.664456339,0.5142,0.3357,0.6005,0.1273,0.1006,0.0797,0.1435,0.1490,5.0157,0f000001,0*ddc696cd\n\tsystem status\tnormal 2 28.000000 0 0\trobot status\t285.776532\t68.893848\t9.962300\t-0.046095\t0.957232\t-29.664456\t0.217000\t0.111000\n\t\n15:23:45.5\tlog_raw\tgps_raw\t#INSPVAXA,USB3,0,48.0,FINESTEERING,2107,282243.550,02000000,471d,15824;INS_ALIGNMENT_COMPLETE,INS_RTKFIXED,37.37075036511,126.72406264733,9.9641,22.3000,-0.1945,0.2497,0.0107,-0.063490953,0.947400713,119.636674206,0.5142,0.3357,0.6005,0.1273,0.1006,0.0797,0.1435,0.1490,5.0157,0f000001,0*2c22af95\n\tsystem status\tnormal 2 28.100000 0 0\trobot status\t285.890404\t68.824275\t9.964100\t-0.063491\t0.947401\t-29.636674\t0.257000\t0.052000\n\t\n15:23:46.0\tlog_raw\tgps_raw\t\tsystem status\tnormal 2 28.000000 0 0\trobot status\t286.004475\t68.753844\t9.966400\t-0.037017\t1.058687\t-29.626598\t0.305000\t-0.012000\n\t\n15:23:46.5\tlog_raw\tgps_raw\t\tsystem status\tnormal 2 28.000000 0 0\trobot status\t286.117617\t68.679949\t9.971000\t0.089227\t1.089857\t-29.625963\t0.295000\t0.002000\n\t\n15:23:47.0\tlog_raw\tgps_raw\t\tsystem status\tnormal 2 28.100000 0 0\trobot status\t286.231219\t68.606305\t9.975700\t0.171162\t1.139452\t-29.676268\t0.293000\t-0.008000\n\t\n15:23:47.5\tlog_raw\tgps_raw\t\tsystem status\tnormal 2 28.000000 0 0\trobot status\t286.345200\t68.531096\t9.979400\t0.265259\t1.249526\t-29.714866\t0.300000\t-0.010000\n\t\n15:23:48.0\tlog_raw\tgps_raw\t\tsystem status\tnormal 2 28.000000 0 0\trobot status\t286.462645\t68.453660\t9.983500\t0.268864\t1.235362\t-29.757203\t0.295000\t-0.015000\n\t\n15:23:48.5\tlog_raw\tgps_raw\t#INSPVAXA,USB3,0,50.0,FINESTEERING,2107,282246.550,02000000,471d,15824;INS_ALIGNMENT_COMPLETE,INS_RTKFIXED,37.37074619554,126.72407050516,9.9901,22.3000,-0.1782,0.2479,0.0044,0.220698175,1.278945577,119.830464589,0.4789,0.3066,0.5774,0.1203,0.0946,0.0781,0.1428,0.1481,5.0182,0f000001,0*b4ea3089\n\tsystem status\tnormal 2 28.100000 0 0\trobot status\t286.586438\t68.361493\t9.990100\t0.220698\t1.278946\t-29.830465\t0.298000\t-0.016000\n\t\n15:23:49.0\tlog_raw\tgps_raw\t\tsystem status\tnormal 2 28.100000 0 0\trobot status\t286.709822\t68.268330\t9.996500\t0.306737\t1.301116\t-29.940455\t0.300000\t-0.016000\n\t\n15:23:49.5\tlog_raw\tgps_raw\t\tsystem status\tnormal 2 28.100000 0 0\trobot status\t286.834150\t68.173362\t10.002800\t0.479429\t1.290014\t-30.090413\t0.298000\t-0.019000\n\t\n15:23:50.0\tlog_raw\tgps_raw\t\tsystem status\tnormal 2 28.100000 0 0\trobot status\t286.958289\t68.080622\t10.008800\t0.514047\t1.298462\t-30.271182\t0.298000\t-0.017000\n\t\n15:23:50.5\tlog_raw\tgps_raw\t\tsystem status\tnormal 2 28.000000 0 0\trobot status\t287.058245\t68.024076\t10.010800\t0.405073\t1.333763\t-30.537943\t0.300000\t-0.014000\n\t\n15:23:51.0\tlog_raw\tgps_raw\t\tsystem status\tnormal 2 28.000000 0 0\trobot status\t287.160015\t67.964977\t10.013000\t0.350726\t1.423059\t-30.814150\t0.298000\t-0.011000\n\t\n15:23:51.5\tlog_raw\tgps_raw\t\tsystem status\tnormal 2 28.000000 0 0\trobot status\t287.282391\t67.873006\t10.018800\t0.427013\t1.514884\t-31.058404\t0.300000\t-0.013000\n\t\n15:23:52.0\tlog_raw\tgps_raw\t\tsystem status\tnormal 2 28.000000 0 0\trobot status\t287.406135\t67.779896\t10.024300\t0.460123\t1.580724\t-31.331818\t0.296000\t-0.012000\n\t\n15:23:52.5\tlog_raw\tgps_raw\t\tsystem status\tnormal 2 28.000000 0 0\trobot status\t287.531615\t67.685849\t10.029000\t0.389150\t1.537280\t-31.624272\t0.296000\t-0.006000\n\t\n15:23:53.0\tlog_raw\tgps_raw\t\tsystem status\tnormal 2 28.100000 0 0\trobot status\t287.652069\t67.594182\t10.032500\t0.464435\t1.490484\t-31.854926\t0.301000\t-0.010000\n\t\n15:23:53.5\tlog_raw\tgps_raw\t\tsystem status\tnormal 2 28.100000 0 0\trobot status\t287.744802\t67.535988\t10.026800\t0.450497\t1.499758\t-32.065314\t0.296000\t-0.003000\n\t\n15:23:54.0\tlog_raw\tgps_raw\t\tsystem status\tnormal 2 28.000000 0 0\trobot status\t287.839361\t67.475891\t10.021800\t0.416745\t1.567074\t-32.273986\t0.298000\t-0.006000\n\t\n15:23:54.5\tlog_raw\tgps_raw\t\tsystem status\tnormal 2 28.100000 0 0\trobot status\t287.946112\t67.398227\t10.021400\t0.440777
